vi "通讯接口数据.vi"(0 "输入-单一更新":T1={"连接方式"=enum."网口(客服端)", "VISA串口名称"="", "服务端识别"={"本机IP"="", "本机端口"=0, "当前目标"="", "服务端侦听ID"=refnum}, "客服端识别"={"客P-主IP:Port"=""}, "ID记录"={}}, 2 "ID记录更新":cluster{"名称":string, "ID":refnum<k5>}, 10 "枚举":T2(ring)) -> (14 "通讯接口数据":T1={"连接方式"=enum."网口(客服端)", "VISA串口名称"="", "服务端识别"={"本机IP"="", "本机端口"=0, "当前目标"="", "服务端侦听ID"=refnum}, "客服端识别"={"客P-主IP:Port"=""}, "ID记录"={}})   [LabVIEW 2019, in "MainPage.lvlib" / "MainPage.lvclass"]
uses:
  MainPage.lvclass
panel:
  # "初始化\n连接方式更改\n串口更改\n服务端识别更改\n客服端识别更改\nID记录更改\nID记录重置"
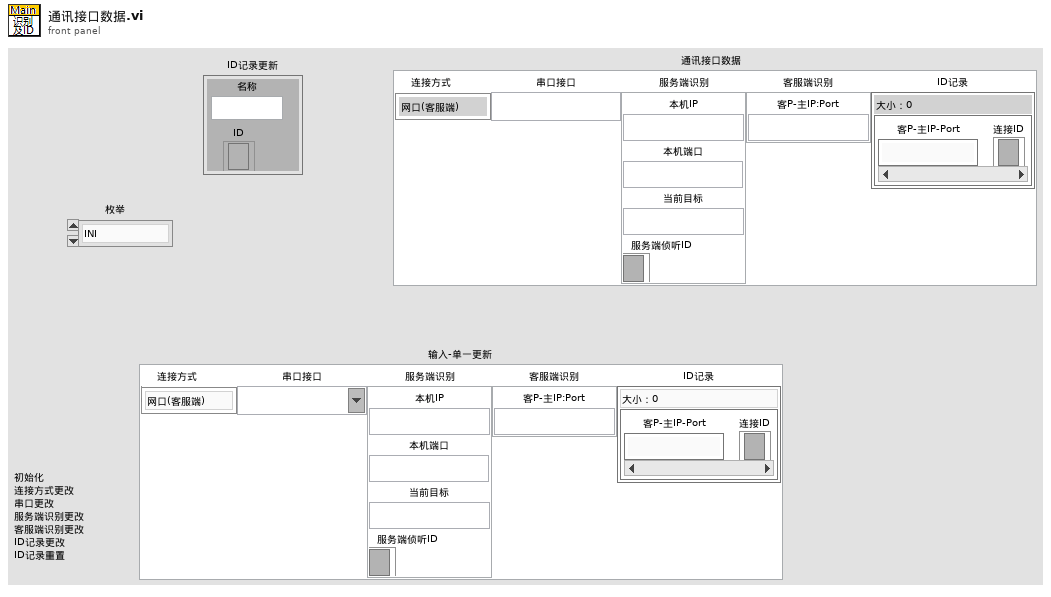
[diagram p1: front panel]
types:
  T1 = typedef "MainPage.lvlib/MainPage.lvclass/DataRef_通讯接口-弃用.ctl" = cluster{"连接方式":enum16{"串口", "网口(客服端)", "网口(服务端)"}, "VISA串口名称":refnum<visa-resource-name>, "服务端识别":cluster{"本机IP":string, "本机端口":u16, "当前目标":string, "服务端侦听ID":refnum<k5>}, "客服端识别":cluster{"客P-主IP:Port":string}, "ID记录":map{string, refnum<k5>}}
  T2 = enum16{"INI", "获取数据", "连接方式更新", "串口更新", "服务端当前目标", "服务端识别及ID", "客服端识别", "ID记录增加", "ID记录删除", "ID记录重置"}
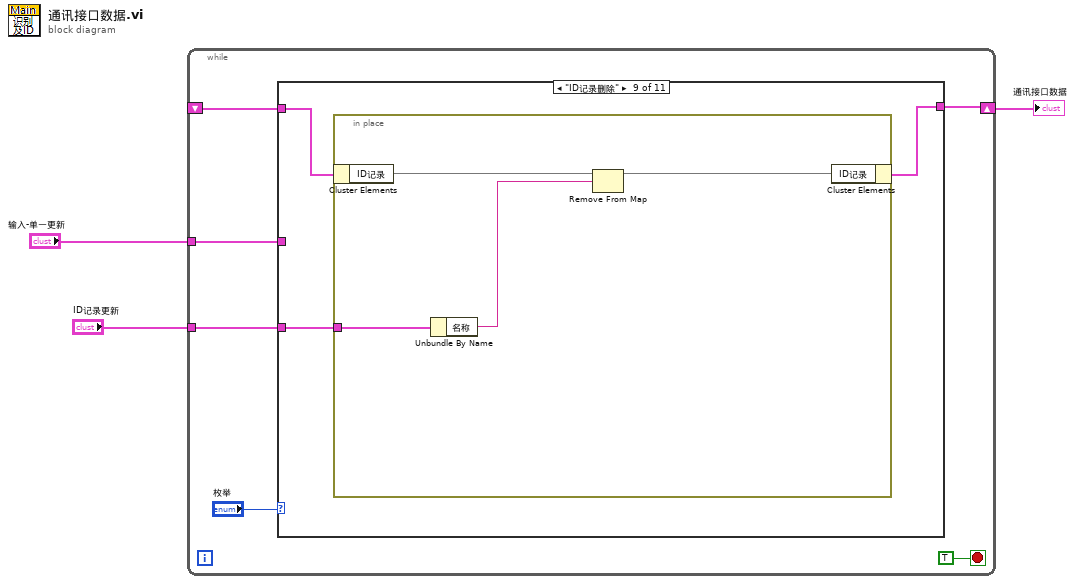
[diagram p0: block diagram]
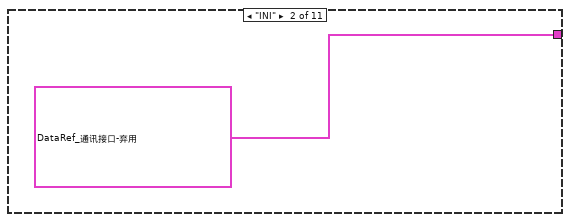
[diagram p3: hidden frame]
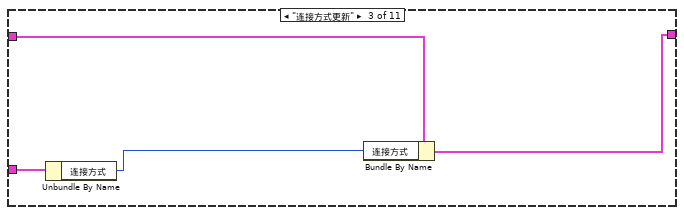
[diagram p4: hidden frame]
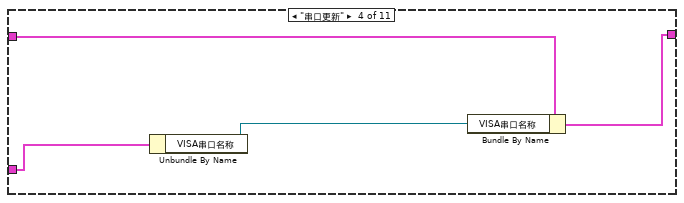
[diagram p5: hidden frame]
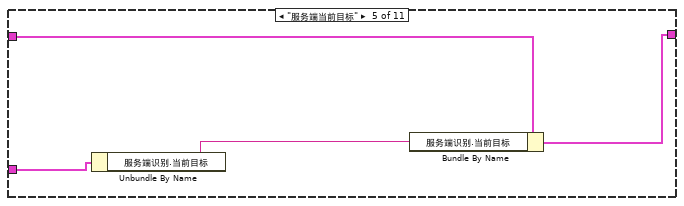
[diagram p6: hidden frame]
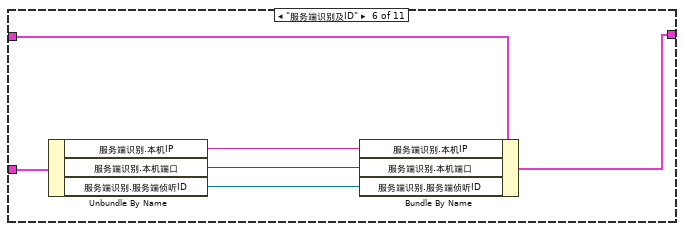
[diagram p7: hidden frame]
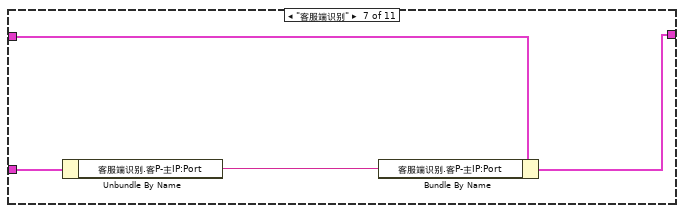
[diagram p8: hidden frame]
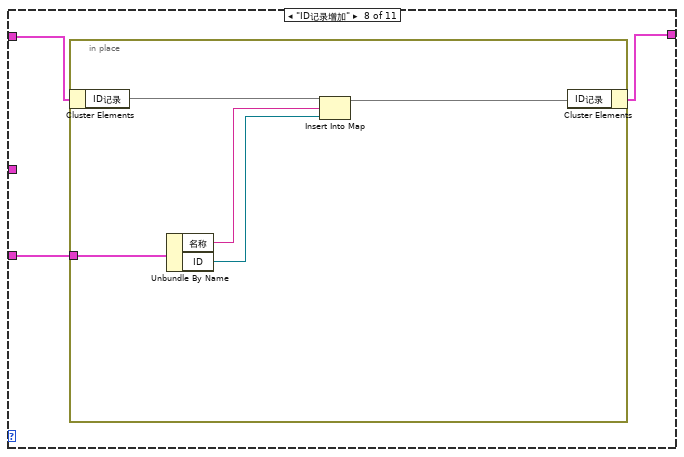
[diagram p9: hidden frame]
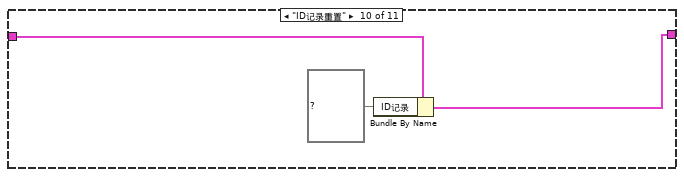
[diagram p10: hidden frame]
diagram:
  n1 = while {
    shift-right: [w7] -> w3
    shift-left: _ -> [w6]
    tunnel: "输入-单一更新" -> [w5]
    tunnel: "ID记录更新" -> [w4]
    stop <- TRUE stop-if-true
    n2 = case shown="\"ID记录删除\"" "枚举" {
      tunnel: [w10 T1 {"连接方式"=enum."串口", "VISA串口名称"="", "服务端识别"={"本机IP"="", "本机端口"=0, "当前目标"="", "服务端侦听ID"=refnum}, "客服端识别"={"客P-主IP:Port"=""}, "ID记录"={}} ("通讯接口数据") w14 w17 w20 w24 w30 w35 w42 w50 w52] -> w7
      tunnel: w6 -> [w10 _ w15 w16 w22 w25 w31 w36 w43 w51 w52]
      tunnel: w5 -> [_ _ w13 w18 w21 w28 w32 _ _ _ _]
      tunnel: w4 -> [_ _ _ _ _ _ _ w34 w44 _ _]
      frame Default {
      }
      frame "INI" {
      }
      frame "连接方式更新" {
        n3 = Unbundle By Name(w13) -> ("连接方式"=w12:enum16{"串口", "网口(客服端)", "网口(服务端)"})
        n4 = Bundle By Name(cluster=w15, "连接方式"=w12) -> (w14:T1)
      }
      frame "串口更新" {
        n5 = Unbundle By Name(w18) -> ("VISA串口名称"=w19:refnum<visa-resource-name>)
        n6 = Bundle By Name(cluster=w16, "VISA串口名称"=w19) -> (w17:T1)
      }
      frame "服务端当前目标" {
        n7 = Unbundle By Name(w21) -> ("服务端识别.当前目标"=w23:string)
        n8 = Bundle By Name(cluster=w22, "服务端识别.当前目标"=w23) -> (w20:T1)
      }
      frame "服务端识别及ID" {
        n9 = Unbundle By Name(w28) -> ("服务端识别.本机IP"=w29:string, "服务端识别.本机端口"=w27:u16, "服务端识别.服务端侦听ID"=w26:refnum<k5>)
        n10 = Bundle By Name(cluster=w25, "服务端识别.本机IP"=w29, "服务端识别.本机端口"=w27, "服务端识别.服务端侦听ID"=w26) -> (w24:T1)
      }
      frame "客服端识别" {
        n11 = Unbundle By Name(w32) -> ("客服端识别.客P-主IP:Port"=w33:string)
        n12 = Bundle By Name(cluster=w31, "客服端识别.客P-主IP:Port"=w33) -> (w30:T1)
      }
      frame "ID记录增加" {
        n13 = in-place {
          in-place-border: w34 -> [w37]
          n14 = in-place-cluster #1(w36) -> ("ID记录"=w41:map{string, refnum<k5>})
          n15 = Unbundle By Name(w37) -> ("名称"=w39:string, "ID"=w38:refnum<k5>)
          n16 = Insert Into Map(map in=w41, key=w39, value=w38) -> (map out=w40:map{string, refnum<k5>})  [unwired: 2 out]
          n17 = in-place-cluster #1("ID记录"=w40) -> (w35:T1)
        }
      }
      frame "ID记录删除" {
        n18 = in-place {
          in-place-border: w44 -> [w47]
          n19 = in-place-cluster #2(w43) -> ("ID记录"=w46:map{string, refnum<k5>})
          n20 = Unbundle By Name(w47) -> ("名称"=w45:string)
          n21 = Remove From Map(10:w45, 11:w46) -> (3:w48:map{string, refnum<k5>})  [unwired: 2 out]
          n22 = in-place-cluster #2("ID记录"=w48) -> (w42:T1)
        }
      }
      frame "ID记录重置" {
        n23 = Bundle By Name(cluster=w51, "ID记录"=map{string, refnum<k5>} {}) -> (w50:T1)
      }
      frame "获取数据" {
      }
    }
  }
  "通讯接口数据" <- w3
